vi "stop.vi"() -> (0 "指令":string)   [LabVIEW 2018]
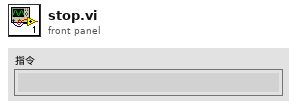
[diagram p1: front panel]
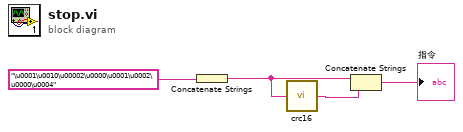
[diagram p0: block diagram]
diagram:
  n1 = Concatenate Strings("\u0001\u0010\u00002\u0000\u0001\u0002\u0000\u0004" ("字符串")) -> (w2:string)
  n2 = call "crc16.vi"("message"=w2) -> ("CRC16"=w3:string)  [unwired: 4 in]
  n3 = Concatenate Strings(w2, w3) -> (→"指令":string)
